vi "Ctor.vi"(8 "error in (no error)":errorcluster) -> (0 "error out":errorcluster, 3 "Class":refnum<class "Recipe Editor.lvclass">)   [LabVIEW 2018, in "Temp Recipe.lvlib" / "Recipe Editor.lvclass"]
uses:
  Recipe Editor.lvclass
  Ref Data.ctl
  Libraries/OOPanel/OOPanel/PanelArray/PanelArray.lvclass
  Update Event Data.ctl
  Libraries/OOPanel/OOPanel/Panel/Panel.lvclass
  Recipe Editor.lvclass/Recipe Editor.ctl
  Temp Recipe.lvlib
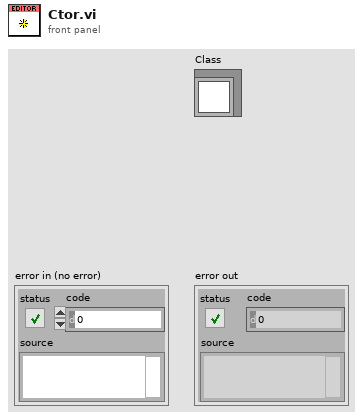
[diagram p1: front panel]
types:
  T1 = typedef "Temp Recipe.lvlib/Update Event Data.ctl" = bool
  T2 = typedef "Temp Recipe.lvlib/Recipe Editor.lvclass/Ref Data.ctl" = cluster{"PanelArray":refnum<class "PanelArray.lvclass">}
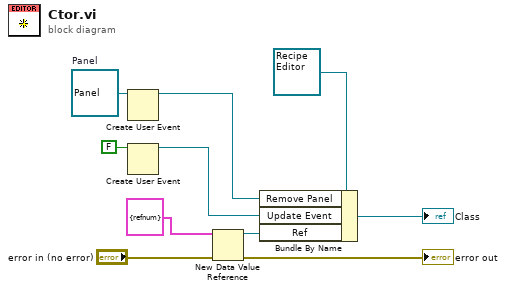
[diagram p0: block diagram]
diagram:
  w2 = refnum<class "Panel.lvclass"> refnum  # Panel
  n1 = Create User Event(user event datatype=w2) -> (user event=w1:refnum<user-event>)  [unwired: 1 in, 1 out]
  n2 = Create User Event(user event datatype=T1 FALSE ("Update")) -> (user event=w4:refnum<user-event>)  [unwired: 1 in, 1 out]
  n3 = New Data Value Reference(data value=T2 {"PanelArray"=refnum} ("Ref Data"), error in="error in (no error)") -> (data value reference=w7:refnum<data-value>, error out=→"error out":errorcluster)
  n4 = Bundle By Name(cluster=refnum<class "Recipe Editor.lvclass"> refnum ("Class In"), "Remove Panel"=w1, "Update Event"=w4, "Ref"=w7) -> (→"Class":refnum<class "Recipe Editor.lvclass">)
